vi "Initialize.vi"(8 "error in (no error)":errorcluster, 10 "Serial Configuration":T1={"Baud Rate "=115200, "Parity "=0, "Data Bits "=8, "Stop Bits"=10} {"Stop Bits" items=["1.0"=10, "1.5"=15, "2.0"=20]; "Data Bits" items=["7"=7, "8"=8]; "Parity" items=["None", "Odd", "Even"]; "Baud Rate" items=["9600"=9600, "19200"=19200, "38400"=38400, "115200"=115200]}, 11 "VISA resource name":refnum<visa-resource-name>) -> (0 "error out":errorcluster, 3 "VISA resource name out":refnum<visa-resource-name>)   [LabVIEW 2021, in "EFD Ultimus V.lvlib"]
doc: "Establishes communication with the Ultimus V. You need to call the Initialize VI only once at the beginning of an application."
uses:
  EFD Ultimus V.lvlib
  <vilib>/Instr/_visa.llb/VISA Configure Serial Port (Instr).vi
panel:
  # "(c) 2009 EFD Inc.  ALL RIGHTS RESERVED."
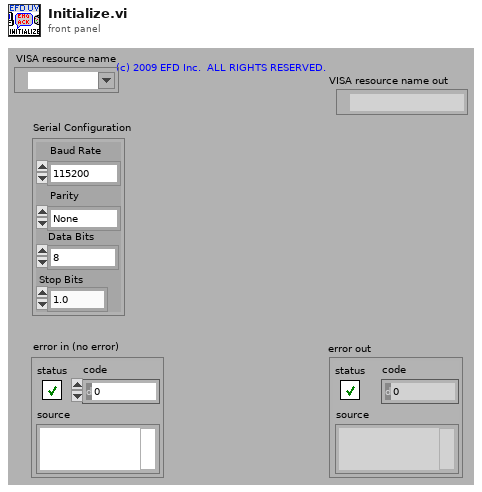
[diagram p1: front panel]
types:
  T1 = cluster{"Baud Rate ":u32, "Parity ":u16, "Data Bits ":u16, "Stop Bits":u16}
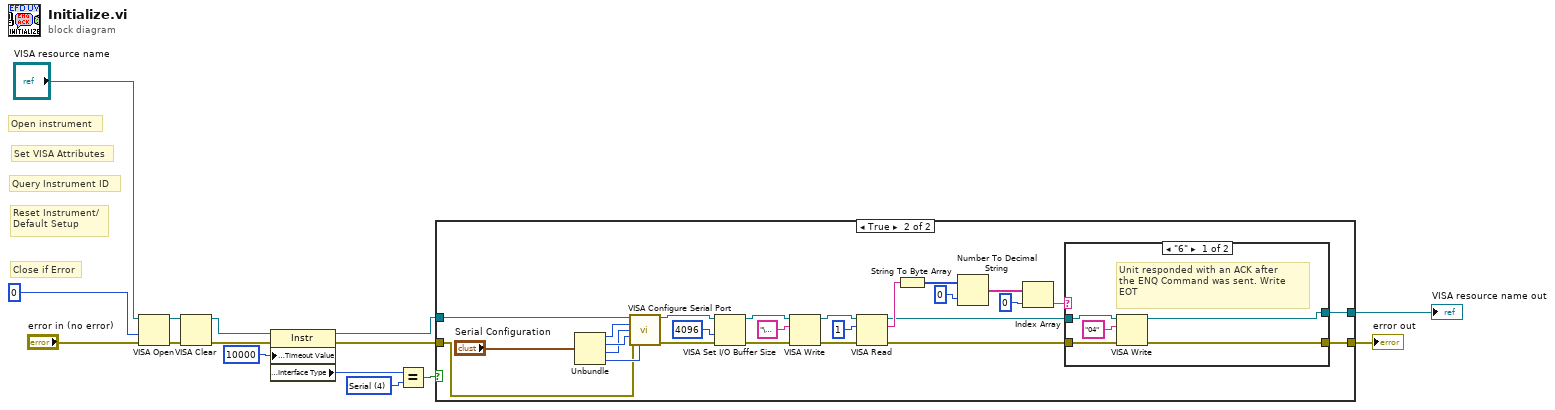
[diagram p0: block diagram]
diagram:
  w8 = u16 4 items=["GPIB"=1, "VXI"=2, "GPIB-VXI"=3, "Serial"=4, "PXI"=5, "TCPIP"=6, "USB"=7] ("Interface Information:Interface Type")
  # "Set VISA Attributes"
  # "Close if Error"
  # "Query Instrument ID"
  # "Reset Instrument/\nDefault Setup"
  # "Open instrument"
  n1 = VISA Open(access mode=u32 0, error in (no error)="error in (no error)", VISA resource name="VISA resource name") -> (VISA resource name=w10:refnum<visa-resource-name>, error out=w11:errorcluster)  [unwired: 2 out]
  n2 = VISA Clear(VISA resource name=w10, error in (no error)=w11) -> (VISA resource name out=w12:refnum<visa-resource-name>, error out=w13:errorcluster)
  n3 = property class="Instr"(reference=w12, error in=w13, "General Settings:Timeout Value"=u32 10000) -> (reference out=w5:refnum<visa-resource-name>, error out=w6:errorcluster, "Interface Information:Interface Type"=w3:u16)
  n4 = Equal?(x=w3, y=w8) -> (x = y?=w7:bool)
  n5 = case shown="True" w7 {
    tunnel: [w16 w19] -> w15
    tunnel: [w17 w21] -> w14
    tunnel: w5 -> [w16 w43]
    tunnel: w6 -> [w17 w18]
    frame False {
    }
    frame True {
      n6 = Unbundle("Serial Configuration") -> ("Baud Rate"=w41:u32, "Parity"=w40:u16, "Data Bits"=w39:u16, "Stop Bits"=w38:u16)
      n7 = call-poly "VISA Configure Serial Port"("VISA resource name"=w43, "baud rate (9600)"=w41, "data bits (8)"=w39, "parity (0:none)"=w40, "error in (no error)"=w18, "stop bits (10: 1 bit)"=w38) -> ("VISA resource name out"=w36:refnum<visa-resource-name>, "error out"=w37:errorcluster)  [unwired: 1 in, 7 out]
      n8 = VISA Set I/O Buffer Size(VISA resource name=w36, size (4096)=u32 4096, error in (no error)=w37) -> (VISA resource name out=w33:refnum<visa-resource-name>, error out=w34:errorcluster)  [unwired: 1 out]
      n9 = VISA Write(VISA resource name=w33, write buffer="\u0005", error in (no error)=w34) -> (VISA resource name out=w30:refnum<visa-resource-name>, error out=w31:errorcluster)  [unwired: 1 out]
      n10 = VISA Read(VISA resource name=w30, byte count=u32 1, error in (no error)=w31) -> (VISA resource name out=w20:refnum<visa-resource-name>, read buffer=w28:string, error out=w22:errorcluster)  [unwired: 1 out]
      n11 = String To Byte Array(string=w28) -> (unsigned byte array=w27:u8[])
      n12 = Number To Decimal String(number=w27, width (-)=i16 0) -> (decimal integer string=w25:string[])
      n13 = Index Array(array=w25, index=0) -> (element=w23:string)
      n14 = case shown="\"6\"" w23 {
        tunnel: w22 -> [w46 w50]
        tunnel: [w45 w50] -> w21
        tunnel: w20 -> [w48 w49]
        tunnel: [w47 w49] -> w19
        frame "6" {
          # "Unit responded with an ACK after\nthe ENQ Command was sent. Write \nEOT"
          n15 = VISA Write(VISA resource name=w48, write buffer="04", error in (no error)=w46) -> (VISA resource name out=w47:refnum<visa-resource-name>, error out=w45:errorcluster)  [unwired: 1 out]
        }
        frame Default {
          # "Error Communicating\nwith the unit, the unit did\nnot reply to the ENQ command"
        }
      }
    }
  }
  "VISA resource name out" <- w15
  "error out" <- w14
